vi "Vision Processing.vi"(4 "error in (no error)":errorcluster) -> ()   [LabVIEW 2018]
doc: "This VI runs in parallel to other tasks. It gets images from the camera, processes them for color or shape and uses commands or globals to affect the behavior of other subsystems."
uses:
  <vilib>/Rock Robotics/WPI/Camera/WPI_CameraImageSize.ctl
  <vilib>/Rock Robotics/WPI/Camera/WPI_CameraFrameRate.ctl
  <vilib>/Rock Robotics/WPI/Camera/WPI_CameraWhite Balance Values.ctl
  <vilib>/Rock Robotics/WPI/Camera/WPI_CameraExposure Values.ctl
  Framework/Robot Global Data.vi
panel:
  in  "Image Size 2":T1=enum."320x240"
  in  "Image Size":T1=enum."320x240"
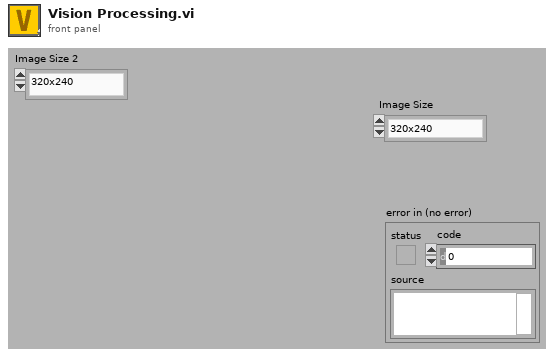
[diagram p1: front panel]
types:
  T1 = typedef "WPI_CameraImageSize.ctl" = enum16{"640x480", "320x240", "160x120", "Custom"}
  T2 = typedef "Image Type" = u32
  T3 = typedef "WPI_CameraExposure Values.ctl" = enum16{"Auto", "Flicker-free 50 Hz", "Flicker-free 60 Hz", "Hold current", "Custom"}
  T4 = typedef "WPI_CameraWhite Balance Values.ctl" = enum16{"Auto", "Fixed indoor", "Fixed outdoor 1", "Fixed outdoor 2", "Fixed fluorescent 1", "Fixed fluorescent 2", "Hold current", "Custom"}
  T5 = typedef "WPI_CameraFrameRate.ctl" = u32
  T6 = typedef "WPI_CameraDevRef.ctl" = cluster{"Camera Address":string, "CameraStatus":errorcluster}
  T7 = typedef "IMAQ Image.ctl" = refnum<image>
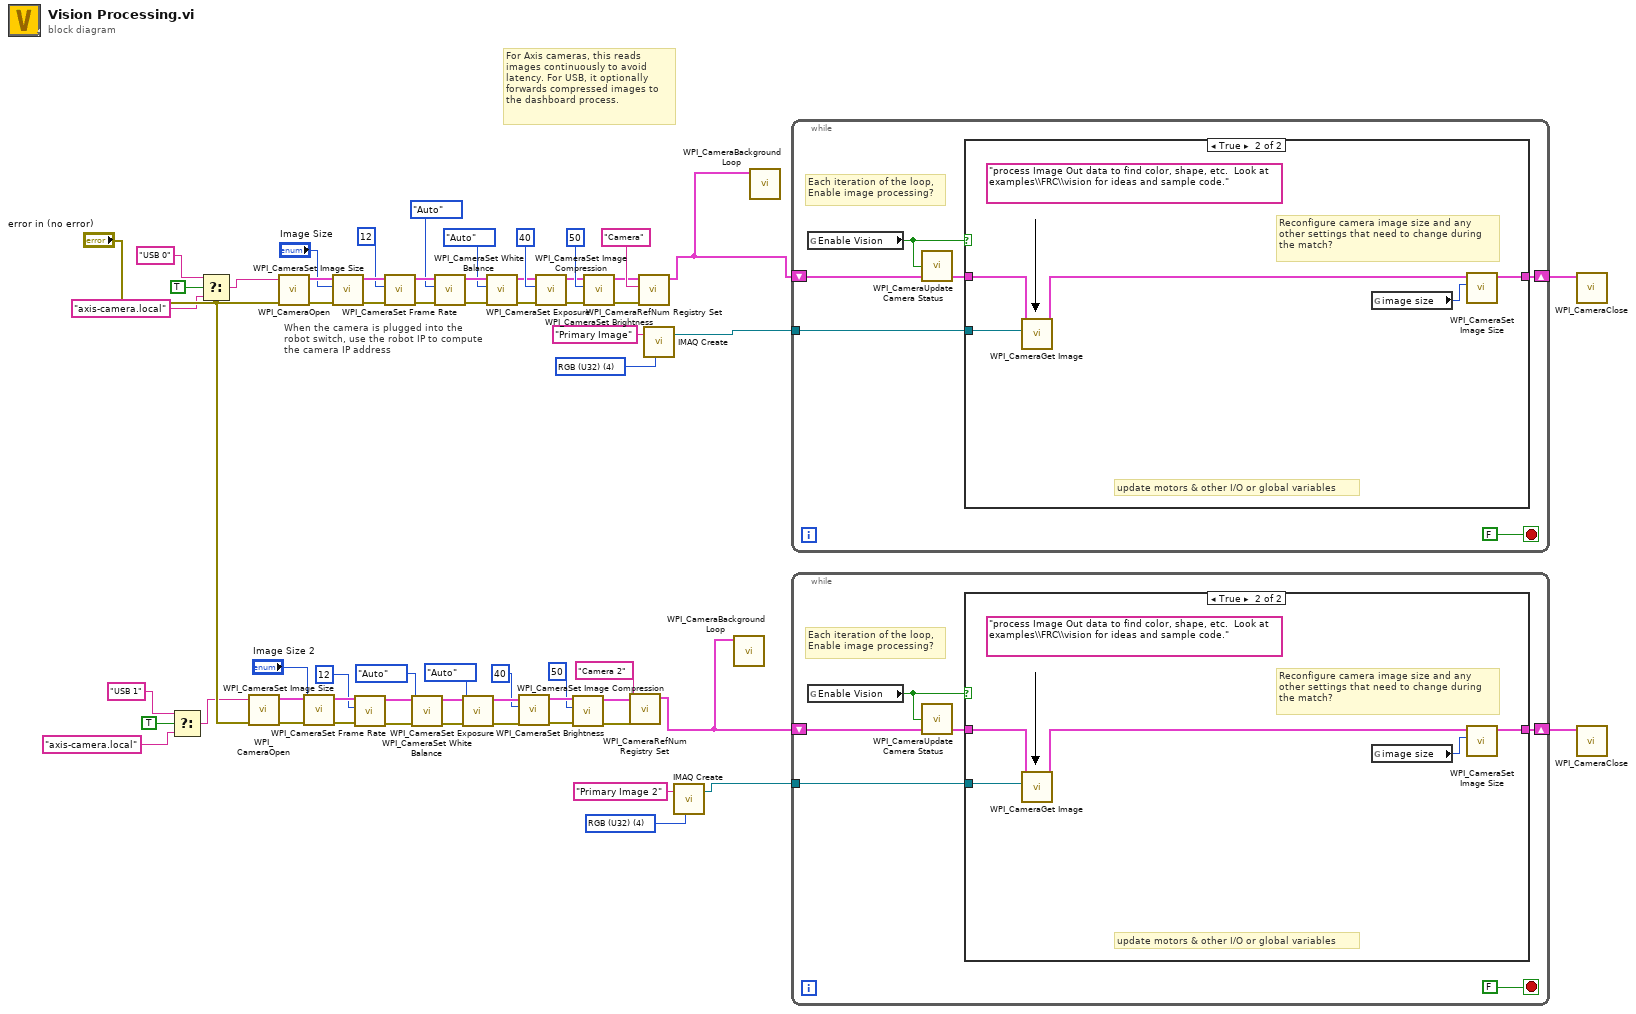
[diagram p0: block diagram]
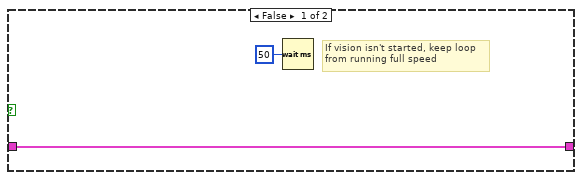
[diagram p2: hidden frame]
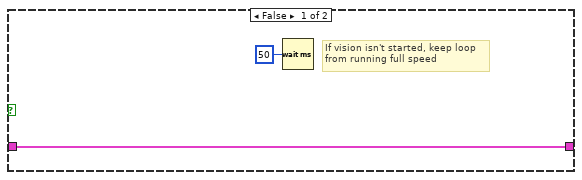
[diagram p3: hidden frame]
diagram:
  w13 = T2 4 items=["Grayscale (U8)", "Grayscale (I16)", "Grayscale (SGL)", "Complex (CSG)", "RGB (U32)", "HSL (U32)", "RGB (U64)"] ("Image Type")
  w61 = T2 4 items=["Grayscale (U8)", "Grayscale (I16)", "Grayscale (SGL)", "Complex (CSG)", "RGB (U32)", "HSL (U32)", "RGB (U64)"] ("Image Type")
  # "When the camera is plugged into the\nrobot switch, use the robot IP to compute\nthe camera IP address"
  # "For Axis cameras, this reads\nimages continuously to avoid\nlatency. For USB, it optionally\nforwards compressed images to\nthe dashboard process."
  n1 = Select(t="USB 1", s=TRUE, f="axis-camera.local") -> (s? t:f=w7:string)
  n2 = Select(t="USB 0", s=TRUE, f="axis-camera.local") -> (s? t:f=w1:string)
  n3 = call <vilib>:"WPI_CameraOpen.vi"("error in (no error)"="error in (no error)", "Camera Address"=w7) -> ("error out"=w36:errorcluster, "CameraDevRef"=w37:T6)  [unwired: 8 in]
  n4 = call <vilib>:"WPI_CameraOpen.vi"("error in (no error)"="error in (no error)", "Camera Address"=w1) -> ("error out"=w49:errorcluster, "CameraDevRef"=w50:T6)  [unwired: 8 out]
  n5 = call <vilib>:"WPI_CameraSet Image Size.vi"("error in (no error)"=w36, "Image Size"="Image Size 2", "CameraDevRef"=w37) -> ("error out"=w35:errorcluster, "CameraDevRef Out"=w34:T6)  [unwired: 7 in]
  n6 = call <vilib>:"WPI_CameraSet Image Size.vi"("error in (no error)"=w49, "Image Size"="Image Size", "CameraDevRef"=w50) -> ("error out"=w48:errorcluster, "CameraDevRef Out"=w51:T6)  [unwired: 1 in, 6 out]
  n7 = call <vilib>:"WPI_CameraSet Frame Rate.vi"("error in (no error)"=w35, "Frame Rate (fps)"=T5 12, "CameraDevRef"=w34) -> ("error out"=w32:errorcluster, "CameraDevRef Out"=w31:T6)  [unwired: 7 in]
  n8 = call <vilib>:"WPI_CameraSet Frame Rate.vi"("error in (no error)"=w48, "Frame Rate (fps)"=T5 12, "CameraDevRef"=w51) -> ("error out"=w47:errorcluster, "CameraDevRef Out"=w53:T6)  [unwired: 7 out]
  n9 = call <vilib>:"WPI_CameraSet White Balance.vi"("error in (no error)"=w32, "White Balance"=WPI_CameraWhite_Balance_Values."Auto", "CameraDevRef"=w31) -> ("error out"=w29:errorcluster, "CameraDevRef Out"=w28:T6)  [unwired: 7 in]
  n10 = call <vilib>:"WPI_CameraSet White Balance.vi"("error in (no error)"=w47, "White Balance"=WPI_CameraWhite_Balance_Values."Auto", "CameraDevRef"=w53) -> ("error out"=w46:errorcluster, "CameraDevRef Out"=w52:T6)  [unwired: 1 in, 6 out]
  n11 = call <vilib>:"WPI_CameraSet Exposure.vi"("error in (no error)"=w29, "Exposure"=WPI_CameraExposure_Values."Auto", "CameraDevRef"=w28) -> ("error out"=w26:errorcluster, "CameraDevRef Out"=w25:T6)  [unwired: 7 in]
  n12 = call <vilib>:"WPI_CameraSet Exposure.vi"("error in (no error)"=w46, "Exposure"=WPI_CameraExposure_Values."Auto", "CameraDevRef"=w52) -> ("error out"=w45:errorcluster, "CameraDevRef Out"=w55:T6)  [unwired: 1 in, 6 out]
  n13 = call <vilib>:"WPI_CameraSet Image Compression.vi"("error in (no error)"=w26, "Compression"=40, "CameraDevRef"=w25) -> ("error out"=w23:errorcluster, "CameraDevRef Out"=w22:T6)  [unwired: 7 in]
  n14 = call <vilib>:"WPI_CameraSet Image Compression.vi"("error in (no error)"=w45, "Compression"=40, "CameraDevRef"=w55) -> ("error out"=w44:errorcluster, "CameraDevRef Out"=w54:T6)  [unwired: 7 out]
  n15 = call <vilib>:"WPI_CameraSet Brightness.vi"("error in (no error)"=w23, "Brightness"=50, "CameraDevRef"=w22) -> ("error out"=w20:errorcluster, "CameraDevRef Out"=w19:T6)  [unwired: 7 in]
  n16 = call <vilib>:"WPI_CameraSet Brightness.vi"("error in (no error)"=w44, "Brightness"=50, "CameraDevRef"=w54) -> ("error out"=w42:errorcluster, "CameraDevRef Out"=w43:T6)  [unwired: 1 in, 6 out]
  n17 = call <vilib>:"WPI_CameraRefNum Registry Set.vi"("error in (no error)"=w20, "refnum name"="Camera 2", "CameraDevRef"=w19) -> ("CameraDevRef"=w9:T6)  [unwired: 7 in, 1 out]
  n18 = call <vilib>:"WPI_CameraRefNum Registry Set.vi"("error in (no error)"=w42, "refnum name"="Camera", "CameraDevRef"=w43) -> ("CameraDevRef"=w10:T6)  [unwired: 1 in, 7 out]
  n19 = call "IMAQ Create"("Image Name"="Primary Image", "Image Type"=w61) -> ("New Image"=w59:T7)  [unwired: 2 in, 2 out]
  n20 = call "IMAQ Create"("Image Name"="Primary Image 2", "Image Type"=w13) -> ("New Image"=w11:T7)  [unwired: 2 in, 2 out]
  n21 = call <vilib>:"WPI_CameraBackground Loop.vi"("CameraDevRef"=w9) -> ()  [unwired: 11 in]
  n22 = call <vilib>:"WPI_CameraBackground Loop.vi"("CameraDevRef"=w10) -> ()  [unwired: 11 in]
  n23 = while {
    shift-right: [w66] -> w38
    shift-left: w10 -> [w64]
    tunnel: w59 -> [w65]
    stop <- FALSE stop-if-true
    # "Each iteration of the loop,\nEnable image processing?"
    n24 = global read "Robot Global Data.vi" "Enable Vision"() -> (w62:bool)
    n25 = call <vilib>:"WPI_CameraUpdate Camera Status.vi"("CameraDevRef In"=w64, "Enable Vision"=w62) -> ("CameraDevRef Out"=w63:T6)  [unwired: 3 in]
    n26 = case shown="True" w62 {
      tunnel: w65 -> [_ w73]
      tunnel: [w69 w74] -> w66
      tunnel: w63 -> [w69 w71]
      frame False {
        # "If vision isn't started, keep loop\nfrom running full speed"
        n27 = Wait (ms)(milliseconds to wait=u32 50) -> ()  [unwired: 1 out]
      }
      frame True {
        (unwired) "process Image Out data to find color, shape, etc.  Look at examples\\FRC\\vision for ideas and sample code."
        # "update motors & other I/O or global variables"
        # "Reconfigure camera image size and any\nother settings that need to change during\nthe match?"
        n28 = call <vilib>:"WPI_CameraGet Image.vi"("Image"=w73, "CameraDevRef"=w71) -> ("CameraDevRef Out"=w70:T6)  [unwired: 1 in, 8 out]
        n29 = global read "Robot Global Data.vi" "image size"() -> (w72:T1)
        n30 = call <vilib>:"WPI_CameraSet Image Size.vi"("Image Size"=w72, "CameraDevRef"=w70) -> ("CameraDevRef Out"=w74:T6)  [unwired: 2 in, 7 out]
      }
    }
  }
  n31 = while {
    shift-right: [w79] -> w14
    shift-left: w9 -> [w77]
    tunnel: w11 -> [w78]
    stop <- FALSE stop-if-true
    # "Each iteration of the loop,\nEnable image processing?"
    n32 = global read "Robot Global Data.vi" "Enable Vision"() -> (w75:bool)
    n33 = call <vilib>:"WPI_CameraUpdate Camera Status.vi"("CameraDevRef In"=w77, "Enable Vision"=w75) -> ("CameraDevRef Out"=w76:T6)  [unwired: 3 in]
    n34 = case shown="True" w75 {
      tunnel: w78 -> [_ w86]
      tunnel: [w82 w87] -> w79
      tunnel: w76 -> [w82 w84]
      frame False {
        # "If vision isn't started, keep loop\nfrom running full speed"
        n35 = Wait (ms)(milliseconds to wait=u32 50) -> ()  [unwired: 1 out]
      }
      frame True {
        (unwired) "process Image Out data to find color, shape, etc.  Look at examples\\FRC\\vision for ideas and sample code."
        # "update motors & other I/O or global variables"
        # "Reconfigure camera image size and any\nother settings that need to change during\nthe match?"
        n36 = call <vilib>:"WPI_CameraGet Image.vi"("Image"=w86, "CameraDevRef"=w84) -> ("CameraDevRef Out"=w83:T6)  [unwired: 1 in, 8 out]
        n37 = global read "Robot Global Data.vi" "image size"() -> (w85:T1)
        n38 = call <vilib>:"WPI_CameraSet Image Size.vi"("Image Size"=w85, "CameraDevRef"=w83) -> ("CameraDevRef Out"=w87:T6)  [unwired: 2 in, 7 out]
      }
    }
  }
  n39 = call <vilib>:"WPI_CameraClose.vi"("CameraDevRef"=w38) -> ()  [unwired: 1 in, 10 out]
  n40 = call <vilib>:"WPI_CameraClose.vi"("CameraDevRef"=w14) -> ()  [unwired: 1 in, 10 out]
